vi "EnqueuePiplelineProcessor.vi"(8 "error in (no error)":errorcluster, 10 "Enqueuer In":T1, 11 "Microscope in":refnum<class "Microscope.lvclass">) -> (0 "error out":errorcluster, 2 "Enqueuer Out":T1, 3 "Microscope out":refnum<class "Microscope.lvclass">)   [LabVIEW 2020, in "Microscope.lvlib" / "Microscope.lvclass"]
uses:
  Microscope.lvclass
  <vilib>/ActorFramework/Message Enqueuer/Message Enqueuer.lvclass
  Microscope.lvclass/Microscope.ctl
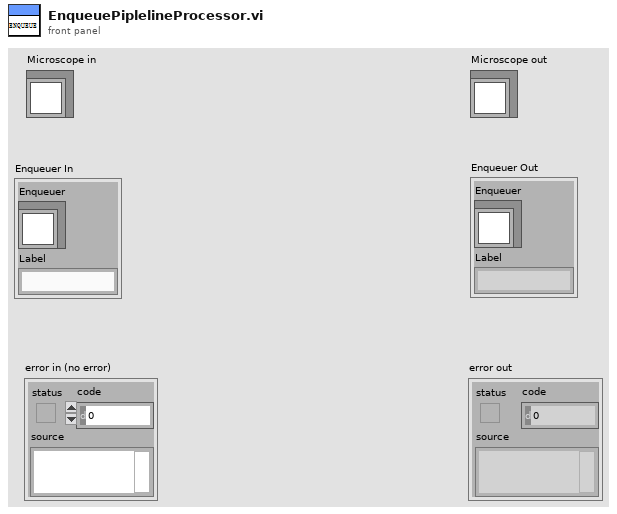
[diagram p1: front panel]
types:
  T1 = cluster{"Enqueuer":refnum<class "Message Enqueuer.lvclass">, "Label":string}
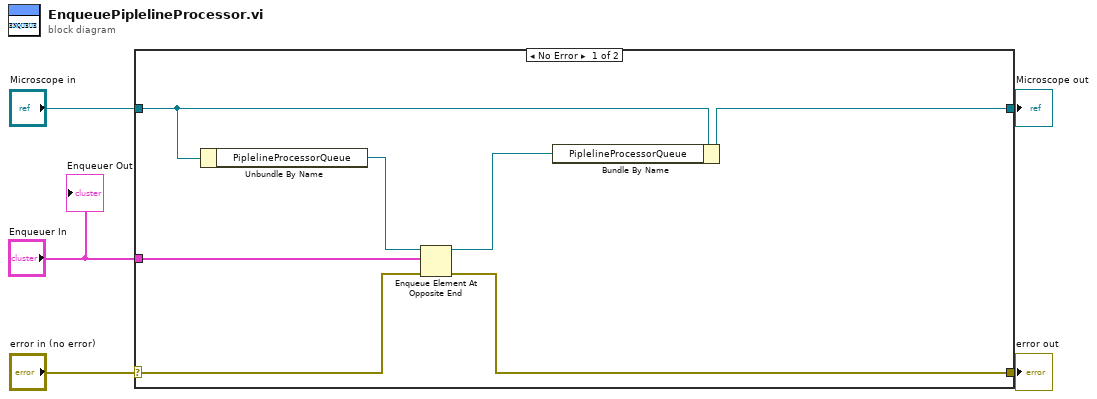
[diagram p0: block diagram]
diagram:
  n1 = case shown="No Error" "error in (no error)" {
    selector: "error in (no error)" -> [w9 w14]
    tunnel: [w8 w14] -> w4
    tunnel: [w10 w13] -> w2
    tunnel: "Microscope in" -> [w12 w13]
    tunnel: "Enqueuer In" -> [w6 _]
    frame No Error {
      n2 = Unbundle By Name(w12) -> ("PiplelineProcessorQueue"=w11:refnum<queue>)
      n3 = Enqueue Element At Opposite End(queue=w11, element=w6, error in (no error)=w9) -> (queue out=w7:refnum<queue>, error out=w8:errorcluster)  [unwired: 1 in, 1 out]
      n4 = Bundle By Name(cluster=w12, "PiplelineProcessorQueue"=w7) -> (w10:refnum<class "Microscope.lvclass">)
    }
    frame Error {
    }
  }
  "error out" <- w4
  "Microscope out" <- w2
  "Enqueuer Out" <- "Enqueuer In"
